vi "Set Slave Info.vi"(7 "Prepend":bool, 8 "error in (no error)":errorcluster, 9 "Slave #":u16, 10 "Slave Name":string, 11 "Item Ref in":T1 format="%.0x") -> (0 "error out":errorcluster, 3 "Item Ref out":T1 format="%.0x")   [LabVIEW 2016, in "Scan Engine Custom Device.lvlib"]
uses:
  Scan Engine Custom Device.lvlib
  <vilib>/NI Veristand/Custom Device API/Custom Device Item Ref.ctl
  Globals/Property Strings.vi
  <vilib>/NI Veristand/Custom Device API/Set Item Property (Boolean).vi
  <vilib>/NI Veristand/Custom Device API/Set Item Property (U16).vi
  <vilib>/NI Veristand/Custom Device API/Custom Device API.lvlib
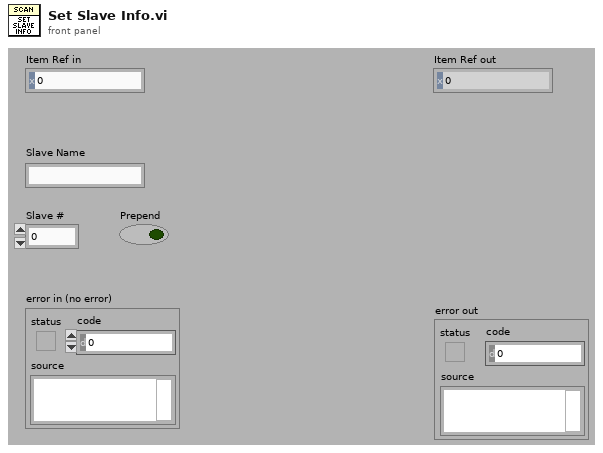
[diagram p1: front panel]
types:
  T1 = typedef "Custom Device API.lvlib/Custom Device Item Ref.ctl" = u64
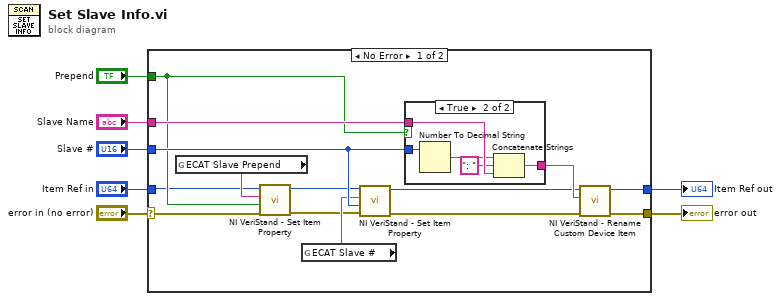
[diagram p0: block diagram]
diagram:
  n1 = case shown="No Error" "error in (no error)" {
    selector: "error in (no error)" -> [w10 w28]
    tunnel: "Item Ref in" -> [w11 w29]
    tunnel: "Slave Name" -> [w20 _]
    tunnel: "Slave #" -> [w19 _]
    tunnel: [w8 w28] -> w3
    tunnel: [w9 w29] -> w2
    tunnel: "Prepend" -> [w15 _]
    frame No Error {
      n2 = global read "Property Strings.vi" "ECAT Slave Prepend"() -> (w14:string)
      n3 = call-poly <vilib>:"NI VeriStand - Set Item Property.vi"("error in (no error)"=w10, "Value"=w15, "Property Name"=w14, "Item Ref in"=w11) -> ("error out"=w13:errorcluster, "Item Ref out"=w12:T1)  [unwired: 5 in, 1 out]
      n4 = global read "Property Strings.vi" "ECAT Slave #"() -> (w16:string)
      n5 = call-poly <vilib>:"NI VeriStand - Set Item Property.vi"("error in (no error)"=w13, "Value"=w19, "Property Name"=w16, "Item Ref in"=w12) -> ("error out"=w18:errorcluster, "Item Ref out"=w17:T1)  [unwired: 5 in, 1 out]
      n6 = case shown="True" w15 {
        tunnel: [w22 w27] -> w21
        tunnel: w20 -> [w22 w26]
        tunnel: w19 -> [_ w25]
        frame False {
        }
        frame True {
          n7 = Number To Decimal String(number=w25) -> (decimal integer string=w24:string)  [unwired: 1 in]
          n8 = Concatenate Strings(w24, ": " ("string"), w26) -> (w27:string)
        }
      }
      n9 = call <vilib>:"NI VeriStand - Rename Custom Device Item.vi"("error in (no error)"=w18, "New Name"=w21, "Item Ref in"=w17) -> ("error out"=w8:errorcluster, "Item Ref out"=w9:T1)  [unwired: 1 in, 6 out]
    }
    frame Error {
    }
  }
  "error out" <- w3
  "Item Ref out" <- w2
